vi "RetrieveTAGprops.vi"(8 "error in (no error)":errorcluster, 11 "FAMM in":refnum<class "FAMM.lvclass">) -> (0 "error out":errorcluster, 3 "FAMM out":refnum<class "FAMM.lvclass">)   [LabVIEW 2020, in "Sgraph_lib_V1.lvlib" / "FAMM.lvclass"]
uses:
  FAMM.lvclass
  FAMM.lvclass/FAMM.ctl
  DBAL/DBAL.lvclass
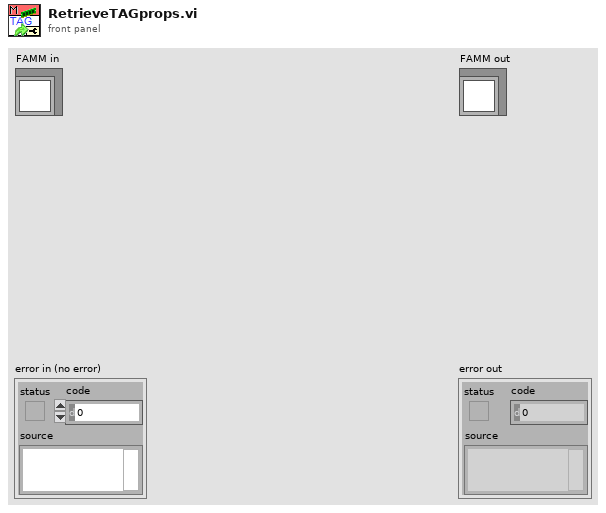
[diagram p1: front panel]
types:
  T1 = typedef "Sgraph_lib_V1.lvlib/FAMM.lvclass/FAMM-attributes.ctl" = cluster{"FAMM_PAQ_Layers":i32, "FAMM_PAQ_resolution":dbl, "PAQ_TAGs":string[], "WAQ_TAGs":string[], "EAQ_TAGs":string[], "All_TAGs":string[], "PAQtagProps":T2[], "WAQtagProps":T2[], "EAQtagProps":T2[], "DBAL_class":refnum<data-value>, "PAQ_memory":refnum<data-value>[], "PAQupdates":timestamp[], "FAMM_Size":cluster{"other":i32, "1day":i32, "1week":i32}, "DatabaseFileExtention":string, "DatabaseSaveRate":dbl, "Database_path":path, "DBAL-Queue":refnum<queue>}
  T2 = typedef "typedef_com_TagProp.ctl" = cluster{"Description":string, "EngUnits":string, "RangeH":dbl, "RangeL":dbl, "Resolution":i32, "Obsolete":bool, "ChangeDate":timestamp, "ChangeSource":string, "ChangeReason":string, "TagFunc":u32}
  T3 = typedef "DBAL_TAGprops.ctl" = T4[]
  T4 = typedef "DBAL_TAGpropEdit.ctl" = cluster{"TAG":string, "Qtype":string, "TAGprop":T2}
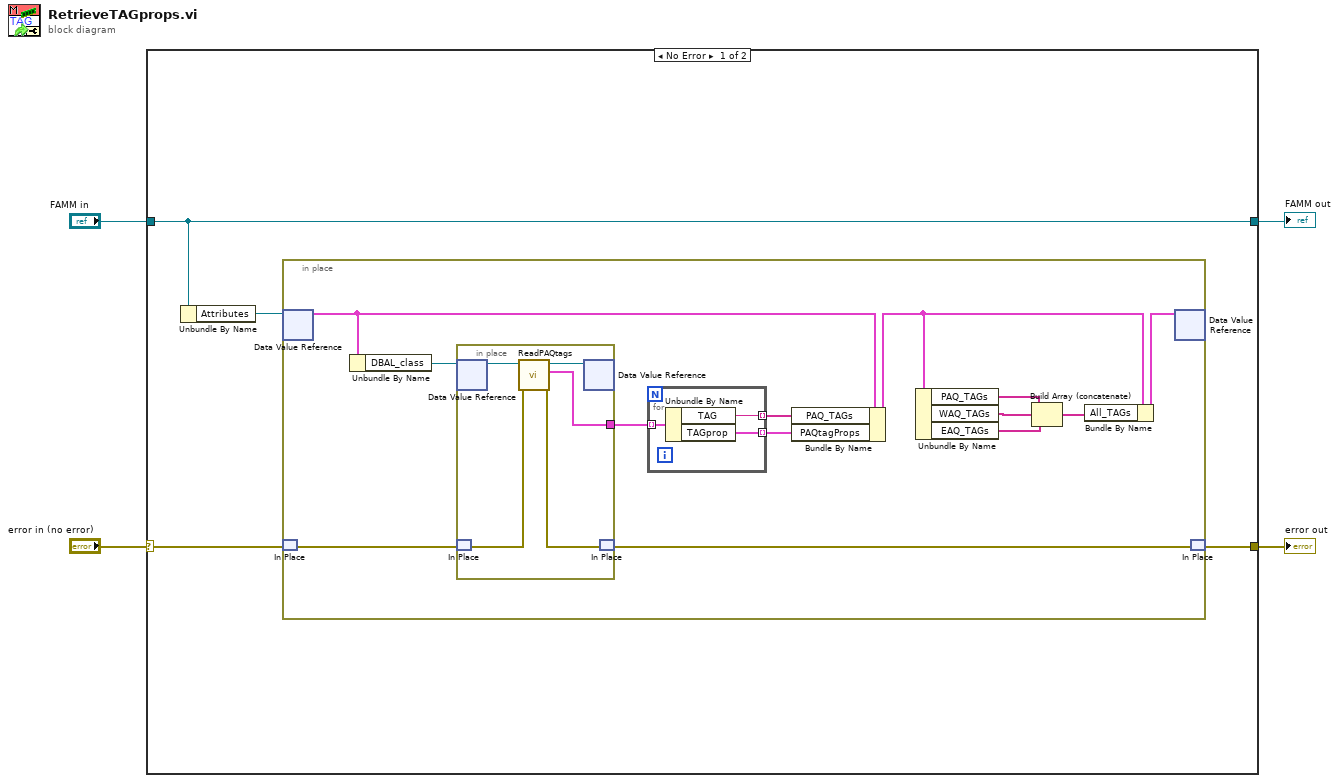
[diagram p0: block diagram]
diagram:
  n1 = case shown="No Error" "error in (no error)" {
    selector: "error in (no error)" -> [w8 w31]
    tunnel: [w7 w31] -> w3
    tunnel: [w6 w30] -> w1
    tunnel: "FAMM in" -> [w6 w30]
    frame No Error {
      n2 = Unbundle By Name(w6) -> ("Attributes"=w5:refnum<data-value>)
      n3 = in-place {
        n4 = in-place-dvr #1(w5) -> (w10:T1)  [unwired: 1 out]
        n5 = in-place-match #2(w8) -> (w13:errorcluster)
        n6 = Unbundle By Name(w10) -> ("DBAL_class"=w11:refnum<data-value>)
        n7 = in-place {
          in-place-border: [w27] -> w16
          n8 = in-place-dvr #3(w11) -> (w26:refnum<class "DBAL.lvclass">)  [unwired: 1 out]
          n9 = in-place-match #4(w13) -> (w29:errorcluster)
          n10 = call-dynamic "ReadPAQtags.vi"("error in (no error)"=w29, "DBAL in"=w26) -> ("error out"=w28:errorcluster, "PAQ_TAGs"=w27:T3, "DBAL out"=w25:refnum<class "DBAL.lvclass">)  [unwired: 7 in]
          n11 = in-place-dvr #3(w25) -> ()  [unwired: 2 out]
          n12 = in-place-match #4(w28) -> (w12:errorcluster)
        }
        n13 = for {
          tunnel: w16 -> [w24] mode=indexing
          tunnel: [w23] -> w15 mode=indexing
          tunnel: [w22] -> w14 mode=indexing
          n14 = Unbundle By Name(w24) -> ("TAG"=w23:string, "TAGprop"=w22:T2)
        }
        n15 = Bundle By Name(cluster=w10, "PAQ_TAGs"=w15, "PAQtagProps"=w14) -> (w9:T1)
        n16 = Unbundle By Name(w9) -> ("PAQ_TAGs"=w21:string[], "WAQ_TAGs"=w20:string[], "EAQ_TAGs"=w19:string[])
        n17 = Build Array (concatenate)(w21, w20, w19) -> (w18:string[])
        n18 = Bundle By Name(cluster=w9, "All_TAGs"=w18) -> (w17:T1)
        n19 = in-place-dvr #1(w17) -> ()  [unwired: 2 out]
        n20 = in-place-match #2(w12) -> (w7:errorcluster)
      }
    }
    frame Error {
    }
  }
  "error out" <- w3
  "FAMM out" <- w1
